vi "FGV Bool.vi"(2 "error in (no error)":errorcluster, 3 "Init/Read/Write State":T1=enum."Write", 4 "Input Node":bool) -> (0 "error out":errorcluster, 1 "Output node":bool)   [LabVIEW 2018]
uses:
  Labview Training Phase 2/Enum Controls/States for Action Engine.ctl
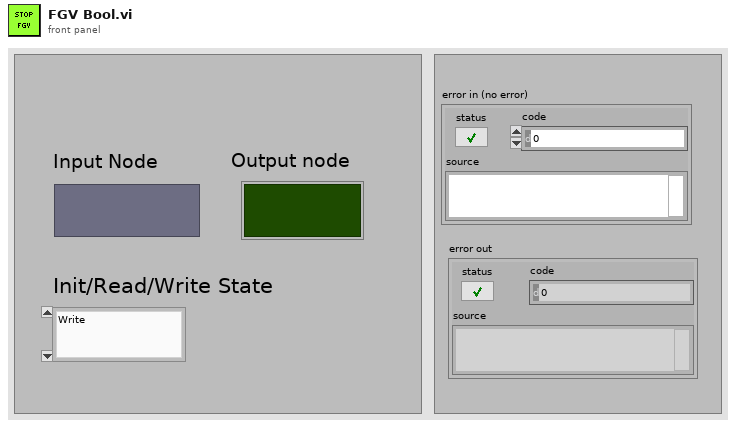
[diagram p1: front panel]
types:
  T1 = typedef "States for Action Engine.ctl" = enum16{"Initialize", "Write", "Read"}
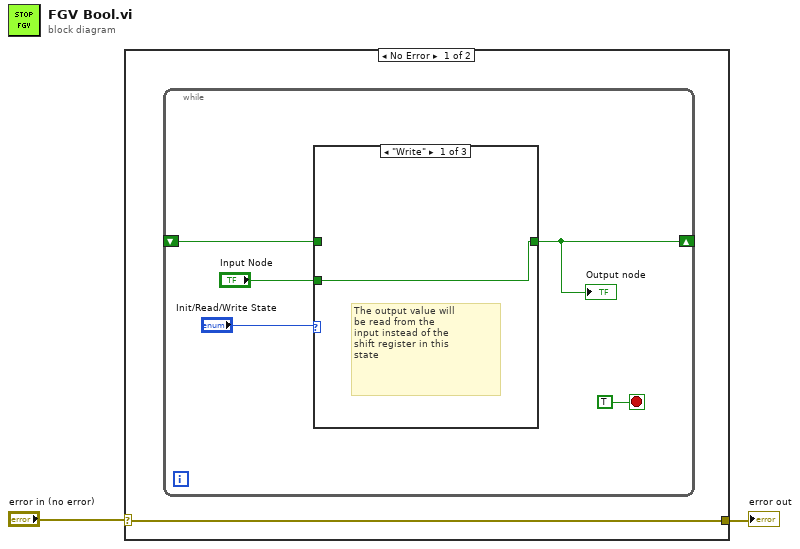
[diagram p0: block diagram]
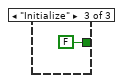
[diagram p3: hidden frame]
diagram:
  n1 = case shown="No Error" "error in (no error)" {
    selector: "error in (no error)" -> [w3 w12]
    tunnel: [w3 w12] -> w1
    frame No Error {
      n2 = while {
        shift-right: [w4] -> _
        shift-left: _ -> [w5]
        stop <- TRUE stop-if-true
        n3 = case shown="\"Write\"" "Init/Read/Write State" {
          tunnel: [w9 w10 FALSE ("Input Node")] -> w4
          tunnel: "Input Node" -> [w9 _ _]
          tunnel: w5 -> [_ w10 _]
          frame "Write" {
            # "The output value will\nbe read from the \ninput instead of the \nshift register in this\nstate"
          }
          frame "Read", Default {
            # "In this state, the output \nvalue is read from \nthe shift register"
          }
          frame "Initialize" {
          }
        }
        "Output node" <- w4
      }
    }
    frame Error {
    }
  }
  "error out" <- w1
